vi "Global 1.vi"() -> ()   [LabVIEW 2024]
panel:
  in  "G-Stop":bool
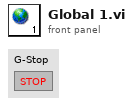
[diagram p1: front panel]
diagram:
